vi "JSON Unflatten Version.vi"(8 "error in (no error)":errorcluster, 11 "version json":string) -> (0 "error out":errorcluster, 3 "version":T1)   [LabVIEW 2017, in "DSF Core.lvlib" / "Configuration Session.lvclass"]
uses:
  Configuration Session.lvclass
  Typedefs/DSF Version Info.ctl
  DSF Core.lvlib
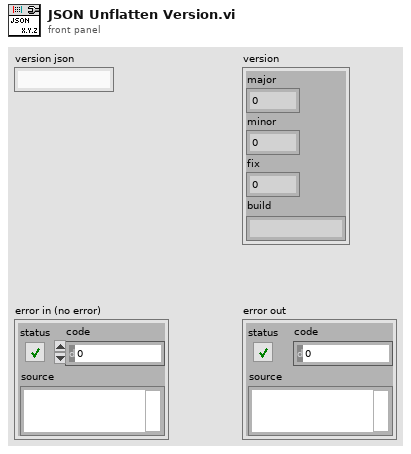
[diagram p1: front panel]
types:
  T1 = typedef "DSF Core.lvlib/DSF Version Info.ctl" = cluster{"major":u32, "minor":u32, "fix":u32, "build":string}
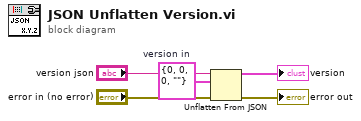
[diagram p0: block diagram]
diagram:
  w2 = T1 {"major"=0, "minor"=0, "fix"=0, "build"=""}  # version in
  n1 = Unflatten From JSON(JSON string="version json", type and defaults=w2, error in (no error)="error in (no error)") -> (value=→"version":T1, error out=→"error out":errorcluster)  [unwired: 4 in]
